vi "GetData.vi"(8 "error in (no error)":errorcluster, 11 "Behavior in":refnum<class "BehaviorData.lvclass">) -> (0 "error out":errorcluster, 1 "Samples":dbl, 2 "data":waveform(dbl)[](array[waveform]), 3 "Behavior out":refnum<class "BehaviorData.lvclass">)   [LabVIEW 2010]
uses:
  <vilib>/DAQmx/read.llb/DAQmx Read (Analog 1D Wfm NChan NSamp).vi
  Program Files/National Instruments/LabVIEW 2010/resource/objmgr/daqmx.rc
  BehaviorData.lvclass
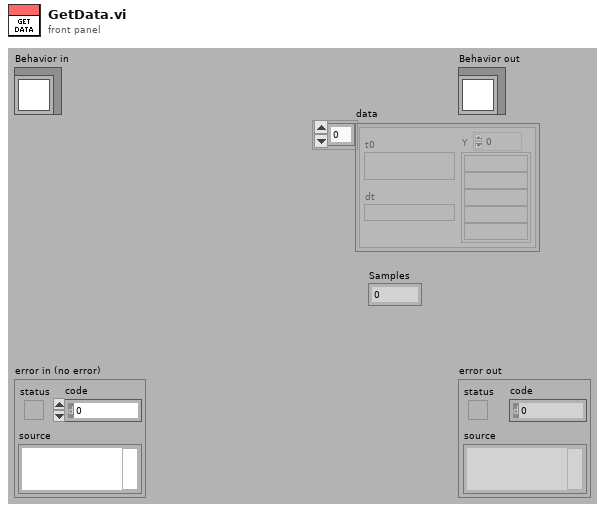
[diagram p1: front panel]
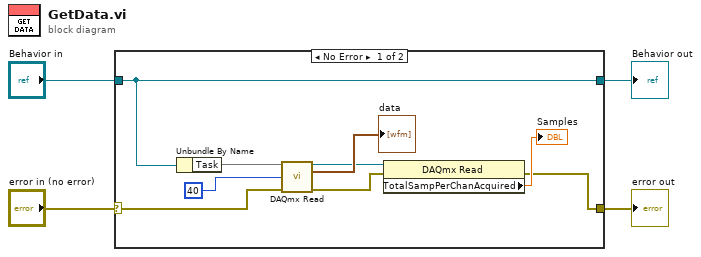
[diagram p0: block diagram]
diagram:
  n1 = case shown="No Error" "error in (no error)" {
    selector: "error in (no error)" -> [w10 w15]
    tunnel: [w5 w15] -> w3
    tunnel: [w13 w14] -> w1
    tunnel: "Behavior in" -> [w13 w14]
    frame No Error {
      n2 = Unbundle By Name(w13) -> ("Task"=w11)
      n3 = call-poly <vilib>:"DAQmx Read.vi"("task/channels in"=w11, "number of samples per channel"=40, "error in"=w10) -> ("task out"=w7:refnum<k21>, "data"=→"data":waveform(dbl)[], "error out"=w6:errorcluster)  [unwired: 10 in]
      n4 = property class="DAQmx Read"(reference=w7, error in=w6) -> (error out=w5:errorcluster, "TotalSampPerChanAcquired"=→"Samples":dbl)  [unwired: 1 out]
    }
    frame Error {
    }
  }
  "error out" <- w3
  "Behavior out" <- w1
